vi "Untitled 1.vi"() -> ()   [LabVIEW 2015]
panel:
  in  "Tree":string(tree)
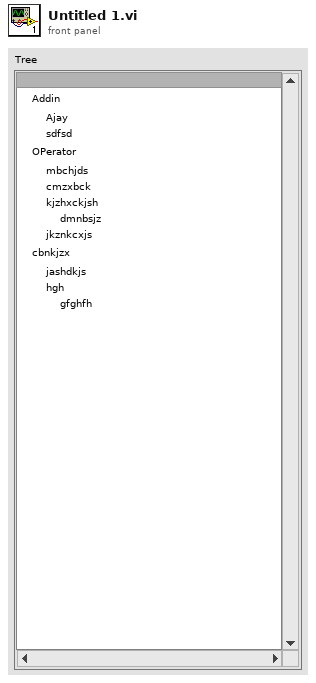
[diagram p1: front panel]
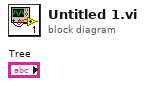
[diagram p0: block diagram]
diagram:
